vi "RunMeas.vi"(8 "error in (no error)":errorcluster, 11 "ChromaPowerSupply in":refnum<class "ChromaPowerSupply.lvclass">) -> (0 "error out":errorcluster, 2 "variant":variant, 3 "ChromaPowerSupply out":refnum<class "ChromaPowerSupply.lvclass">)   [LabVIEW 2018, in "AcPwrPlugins.lvlib" / "ChromaPowerSupply.lvclass"]
doc: "This VI initiates and takes measurements from the instrument(s)."
uses:
  ChromaPowerSupply.lvclass
  AcPwrShared/clMeasurmentData.ctl
  AcPwrShared/clAcPwrAttributes.ctl
  AcPwrShared/AcPwrShared.lvlib
  ChromaAcLoad/ChromaAcLoad.lvclass
panel:
  out "Waveform Chart":waveform(dbl)[](graph)
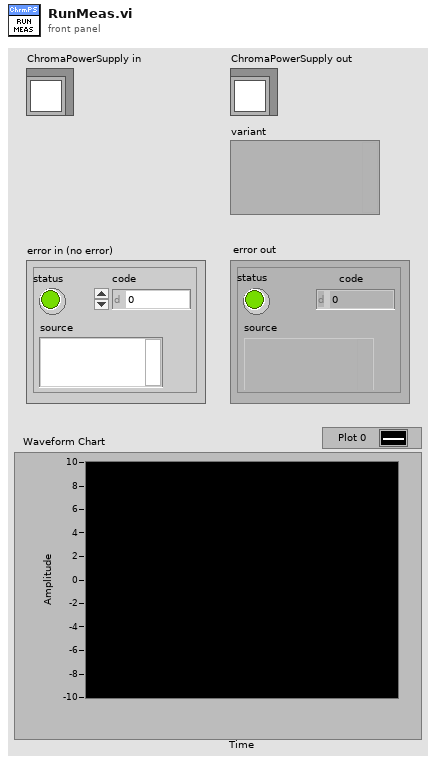
[diagram p1: front panel]
types:
  T1 = typedef "AcPwrPlugins.lvlib/ChromaPowerSupply.lvclass/Measurements.ctl" = cluster{"Handle":string, "Name":string, "Enabled":bool, "Measurement Value":dbl, "btnMeasFetch":bool, "ProtectionStatusString":string, "Measurement Type":enum16{"Voltage (V)", "Current (A)", "Power (W)"}}[]
  T2 = typedef "AcPwrPlugins.lvlib/ChromaPowerSupply.lvclass/Device(s)Settings.ctl" = cluster{"Phases":cluster{"Handle":string, "Instrument Options":string, "id query (T)":bool, "reset device (T)":bool, "Timing":cluster{"TimingOn":enum16{""}, "Hours":u32, "Minutes":u32, "Seconds":dbl, "CutoffVoltage":dbl}, "Connected":bool, "Output Mode":enum16{"Voltage (DC)", "Current (DC)"}, "Voltage":dbl, "Current":dbl, "Voltage Limit":dbl, "Current Limit":dbl}[], "MeasName":string}
  T3 = typedef "AcPwrShared.lvlib/clMeasurmentData.ctl" = cluster{"MeasName":string, "XML Data":string, "WaveformData":waveform(dbl)[]}
  T4 = typedef "AcPwrShared.lvlib/clAcPwrAttributes.ctl" = cluster{"ProtectionStatusString":string, "Handle_MeasurementType":string, "Status Byte Register":cluster{"Busy":bool, "Remote Mode":bool, "Error in Queue":bool, "QUES=Questionable Status Summary":bool, "MAV = Message Available":bool, "ESB = Event Status Byte Summary":bool, "RQS = Request for Service":bool, "OPER = Operation Event Summary":bool}}
  T5 = enum16{"Voltage (V)", "Current (A)", "Power (W)"}
  T6 = cluster{"Handle":string, "Name":string, "Enabled":bool, "Measurement Value":dbl, "btnMeasFetch":bool, "ProtectionStatusString":string, "Measurement Type":enum16{"Voltage (V)", "Current (A)", "Power (W)"}}
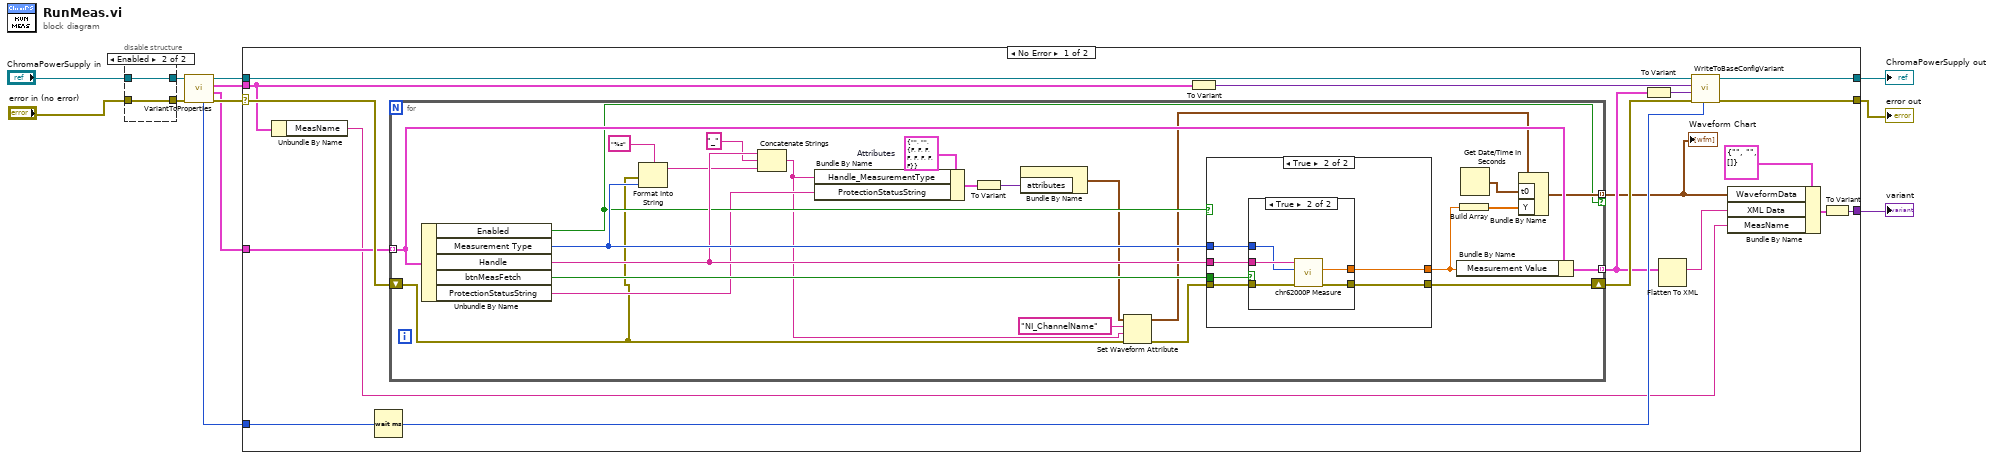
[diagram p0: block diagram]
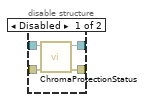
[diagram p2: hidden frame]
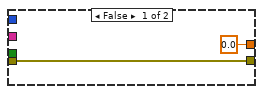
[diagram p3: hidden frame]
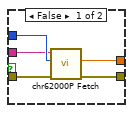
[diagram p4: hidden frame]
diagram:
  n1 = disable-structure shown="Enabled" {
    disable-tunnel: [w16 w17] -> w12
    disable-tunnel: [w15 w18] -> w11
    disable-tunnel: "ChromaPowerSupply in" -> [w14 w18]
    disable-tunnel: "error in (no error)" -> [w13 w17]
    frame Disabled {
      n2 = call "ChromaProtectionStatus.vi"("error in (no error)"=w13, "ChromaAcLoad in"=w14) -> ("error out"=w16:errorcluster, "ChromaAcLoad out"=w15:refnum<class "ChromaAcLoad.lvclass">)  [unwired: 8 in]
    }
    frame Enabled {
    }
  }
  n3 = call-dynamic "VariantToProperties.vi"("error in (no error)"=w12, "ChromaPowerSupply in"=w11) -> ("error out"=w7:errorcluster, "Measurements"=w6:T1, "Device Settings"=w5:T2, "ChromaPowerSupply out"=w9:refnum<class "ChromaPowerSupply.lvclass">, "Measurement Refresh Time (ms)"=w4:u32)  [unwired: 5 in]
  n4 = case shown="No Error" w7 {
    selector: w7 -> [w36 w79]
    tunnel: [w32 w80] -> w3
    tunnel: [w30 w79] -> w1
    tunnel: w9 -> [w34 w80]
    tunnel: w5 -> [w27 _]
    tunnel: w6 -> [w35 _]
    tunnel: w4 -> [w28 _]
    tunnel: [w20 _] -> w2
    frame No Error {
      n5 = Unbundle By Name(w27) -> ("MeasName"=w21:string)
      n6 = Wait (ms)(milliseconds to wait=w28) -> (millisecond timer value=w26:u32)
      n7 = for {
        tunnel: w35 -> [w60] mode=indexing
        shift-right: [w58] -> w33
        shift-left: w36 -> [w37]
        tunnel: [w59] -> w25 mode=indexing
        tunnel: [w54] -> w19 mode=indexing if=w46
        w45 = T4 {"ProtectionStatusString"="", "Handle_MeasurementType"="", "Status Byte Register"={"Busy"=FALSE, "Remote Mode"=FALSE, "Error in Queue"=FALSE, "QUES=Questionable Status Summary"=FALSE, "MAV = Message Available"=FALSE, "ESB = Event Status Byte Summary"=FALSE, "RQS = Request for Service"=FALSE, "OPER = Operation Event Summary"=FALSE}}  # Attributes
        n8 = Unbundle By Name(w60) -> ("Enabled"=w46:bool, "Measurement Type"=w51:T5, "Handle"=w49:string, "btnMeasFetch"=w57:bool, "ProtectionStatusString"=w43:string)
        n9 = Format Into String(format string="%s", error in=w37, w51) -> (resulting string=w47:string)  [unwired: 1 in, 1 out]
        n10 = Concatenate Strings(w49, "_", w47) -> (w39:string)
        n11 = Bundle By Name(cluster=w45, "Handle_MeasurementType"=w39, "ProtectionStatusString"=w43) -> (w44:T4)
        n12 = To Variant(anything=w44) -> (Variant=w50:variant)
        n13 = Bundle By Name("attributes"=w50) -> (w38:waveform(dbl))  [unwired: 1 in]
        n14 = Set Waveform Attribute(4:w37, 5:w39, 6:"NI_ChannelName" ("name"), 7:w38) -> (0:w41:errorcluster, 3:w40:waveform(dbl))  [unwired: 1 out]
        n15 = case shown="True" w46 {
          tunnel: w41 -> [w62 w65]
          tunnel: w51 -> [_ w64]
          tunnel: [w62 w66] -> w58
          tunnel: [0.0 ("Query CF of Current") w63] -> w56
          tunnel: w49 -> [_ w67]
          tunnel: w57 -> [_ w68]
          frame False {
          }
          frame True {
            n16 = case shown="True" w68 {
              tunnel: w67 -> [w71 w78]
              tunnel: [w70 w77] -> w66
              tunnel: w65 -> [w73 w76]
              tunnel: w64 -> [w72 w74]
              tunnel: [w69 w75] -> w63
              frame False {
                n17 = call <instrlib>:"chr62000P Fetch.vi"("error in (no error)"=w73, "Fetch Type (Voltage)"=w72, "instrument handle"=w71) -> ("error out"=w70:errorcluster, "ReadValue"=w69:dbl)  [unwired: 6 in, 1 out]
              }
              frame True {
                n18 = call <instrlib>:"chr62000P Measure.vi"("error in (no error)"=w76, "Measure Type (Voltage)"=w74, "instrument handle"=w78) -> ("error out"=w77:errorcluster, "ReadValue"=w75:dbl)  [unwired: 6 in, 1 out]
              }
            }
          }
        }
        n19 = Bundle By Name(cluster=w60, "Measurement Value"=w56) -> (w59:T6)
        n20 = Build Array(w56) -> (w55:dbl[])
        n21 = Get Date/Time In Seconds() -> (seconds since 1Jan1904=w53:timestamp)
        n22 = Bundle By Name(cluster=w40, "t0"=w53, "Y"=w55) -> (w54:waveform(dbl))
      }
      "Waveform Chart" <- w19
      n23 = To Variant(anything=w27) -> (Variant=w29:variant)
      n24 = To Variant(anything=w25) -> (Variant=w31:variant)
      n25 = Flatten To XML(anything=w25) -> (xml string=w22:string)
      n26 = call-dynamic "WriteToBaseConfigVariant.vi"("Measurement Refresh Time (ms)"=w26, "error in (no error)"=w33, "Meas"=w31, "Config"=w29, "ChromaPowerSupply in"=w34) -> ("error out"=w30:errorcluster, "ChromaPowerSupply out"=w32:refnum<class "ChromaPowerSupply.lvclass">)  [unwired: 5 in]
      n27 = Bundle By Name(cluster=T3 {"MeasName"="", "XML Data"="", "WaveformData"=[]} ("MeasurmentDataCluster"), "WaveformData"=w19, "XML Data"=w22, "MeasName"=w21) -> (w23:T3)
      n28 = To Variant(anything=w23) -> (Variant=w20:variant)
    }
    frame Error {
    }
  }
  "ChromaPowerSupply out" <- w3
  "error out" <- w1
  "variant" <- w2
